vi "setUp.vi"(8 "Error in (no error)":errorcluster, 11 "Reference in":refnum<class "Static TestSuite.lvclass">) -> (0 "Error out":errorcluster, 3 "Reference out":refnum<class "Static TestSuite.lvclass">)   [LabVIEW 2013, in "Static TestSuite.lvclass"]
uses:
  Static TestSuite.lvclass
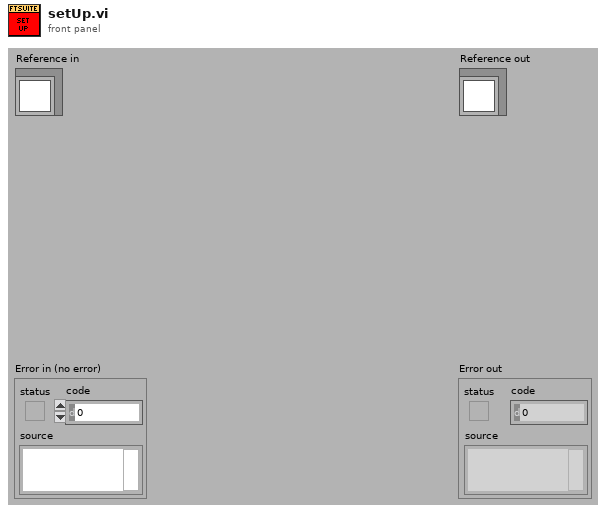
[diagram p1: front panel]
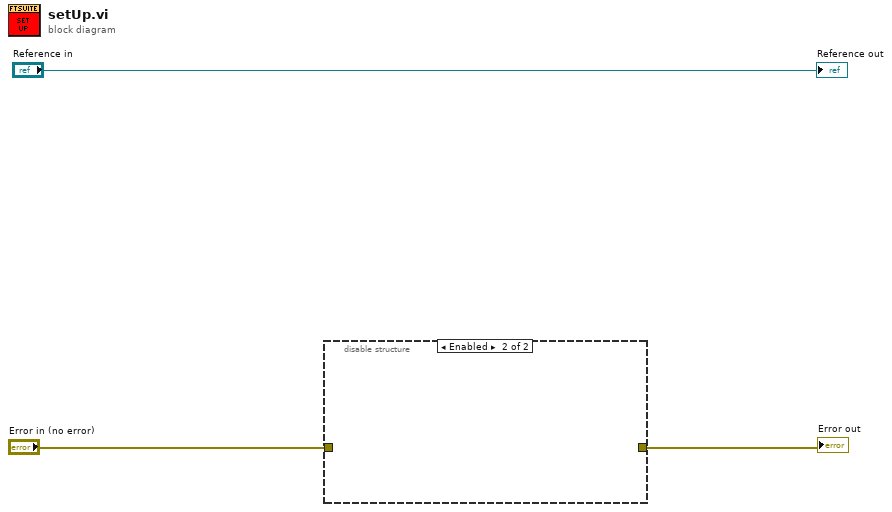
[diagram p0: block diagram]
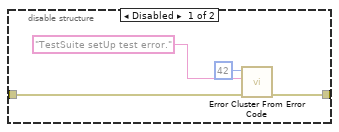
[diagram p2: hidden frame]
diagram:
  n1 = disable-structure shown="Enabled" {
    disable-tunnel: "Error in (no error)" -> [w7 _]
    disable-tunnel: [w6 _] -> w1
    frame Disabled {
      n2 = call <vilib>:"Error Cluster From Error Code.vi"("error in (no error)"=w7, "error message (\"\")"="TestSuite setUp test error." ("error message (\"\")"), "error code (0)"=42) -> ("error out"=w6:errorcluster)  [unwired: 6 in]
    }
    frame Enabled {
    }
  }
  "Error out" <- w1
  "Reference out" <- "Reference in"
